vi "NML AI Waveform Scan.vi"(0 "task/channels in":refnum<k21>, 1 "stop":bool, 2 "Number to Average":i32=128, 5 "error in":errorcluster) -> (6 "task out":refnum<k21>, 7 "Scaled data":dbl[][](array[numeric]) format="%.3e", 8 "error out":errorcluster)   [LabVIEW 2021]
uses:
  <vilib>/_DAQmxBase/Internals/DAQmxBase Read (Analog 2D DBL NChan NSamp).vi
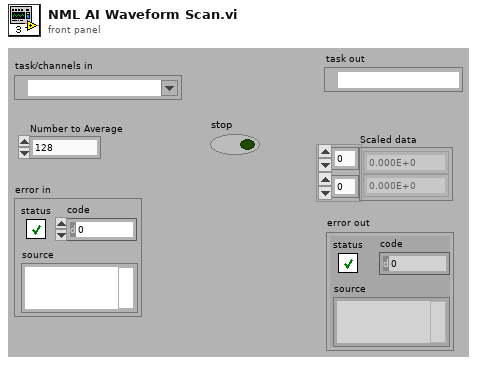
[diagram p1: front panel]
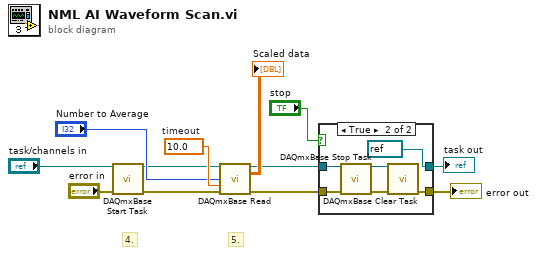
[diagram p0: block diagram]
diagram:
  w11 = 10.0  # timeout
  # "5."
  # "4."
  n1 = call <vilib>:"DAQmxBase Start Task.vi"("task/channels in"="task/channels in", "error in"="error in") -> ("task out"=w9:refnum<k21>, "error out"=w8:errorcluster)  [unwired: 12 in]
  n2 = call-poly <vilib>:"DAQmxBase Read.vi"("task/channels in"=w9, "number of samples per channel"="Number to Average", "timeout"=w11, "error in"=w8) -> ("task out"=w3:refnum<k21>, "data"=→"Scaled data":dbl[][], "error out"=w4:errorcluster)  [unwired: 9 in]
  n3 = case shown="True" "stop" {
    tunnel: [w14 w16] -> w2
    tunnel: w4 -> [w14 w17]
    tunnel: w3 -> [w13 w18]
    tunnel: [w13 refnum<k21> refnum ("task out")] -> w1
    frame False {
    }
    frame True {
      n4 = call <vilib>:"DAQmxBase Stop Task.vi"("task/channels in"=w18, "error in"=w17) -> ("task out"=w20:refnum<k21>, "error out"=w19:errorcluster)  [unwired: 12 in]
      n5 = call <vilib>:"DAQmxBase Clear Task.vi"("task in"=w20, "error in"=w19) -> ("error out"=w16:errorcluster)  [unwired: 13 in]
    }
  }
  "task out" <- w1
  "error out" <- w2
